vi "DIO timeline.vi"(1 "Plot?":bool[][](array[boolean]), 2 "Array":u64[][](array[numeric])=[[0, 51168, 5155], [1000, 51168, 5155], [2000, 50912, 5155], [20000, 49888, 5155], [14960, 49888, 5155], [16960, 49888, 5155], [17960, 49888, 5155], [31420, 49376, 5155], [33920, 49376, 5153], [50880, 49376, 5139], [62840, 50656, 5139], [1304, 50592, 5139], [2304, 50592, 5139], [3304, 50656, 5139], [4304, 50400, 5139], [22304, 49376, 5139], [38552, 50656, 5139], [42552, 50592, 5139], [43552, 50592, 5139], [44552, 50656, 5139], [45552, 50400, 5139], [63552, 49376, 5139], [19264, 49888, 5155], [60512, 49888, 5155], [34224, 49888, 5155], [36224, 49888, 5153], [50184, 49888, 5153], [50684, 49896, 5153], [51184, 49864, 5281], [53184, 49866, 13473], [53384, 33482, 13473], [53534, 33482, 13473], [53584, 49866, 13473], [53684, 49864, 13473], [54184, 49864, 13345], [55184, 49856, 13345], [58184, 49856, 5153], [4608, 49857, 5153], [16568, 51137, 5153], [19568, 51137, 7201], [20568, 51105, 7201], [21568, 50996, 7201], [21668, 51120, 7201], [22568, 51184, 7201], [23068, 51168, 7201], [23568, 50912, 7201], [31568, 50912, 5153], [41568, 49888, 5153], [57816, 51168, 5153], [60816, 51168, 7201], [61816, 51104, 7201], [62816, 50996, 7201], [62916, 51120, 7201], [63816, 51184, 7201], [64316, 51168, 7201], [64816, 50912, 7201], [7280, 50912, 5153], [17280, 49888, 5153], [33528, 51168, 5153], [37528, 51104, 5153], [39528, 51168, 5153], [40528, 50912, 5153], [58528, 49888, 5153], [14240, 49888, 5155]]) -> (0 "Timeline":cluster{u32[], i32[]}[](graph))   [LabVIEW 2017]
uses:
  globals/DIO board parameters global.vi
panel:
  out "Array 2":cluster{u32[], u32[]}[](array[cluster])
  # "00  01  02  03  04  05  06  07  08  09  10  11  12  13  14  15"
  # "Port A\nPort B\nPort C\nPort D"
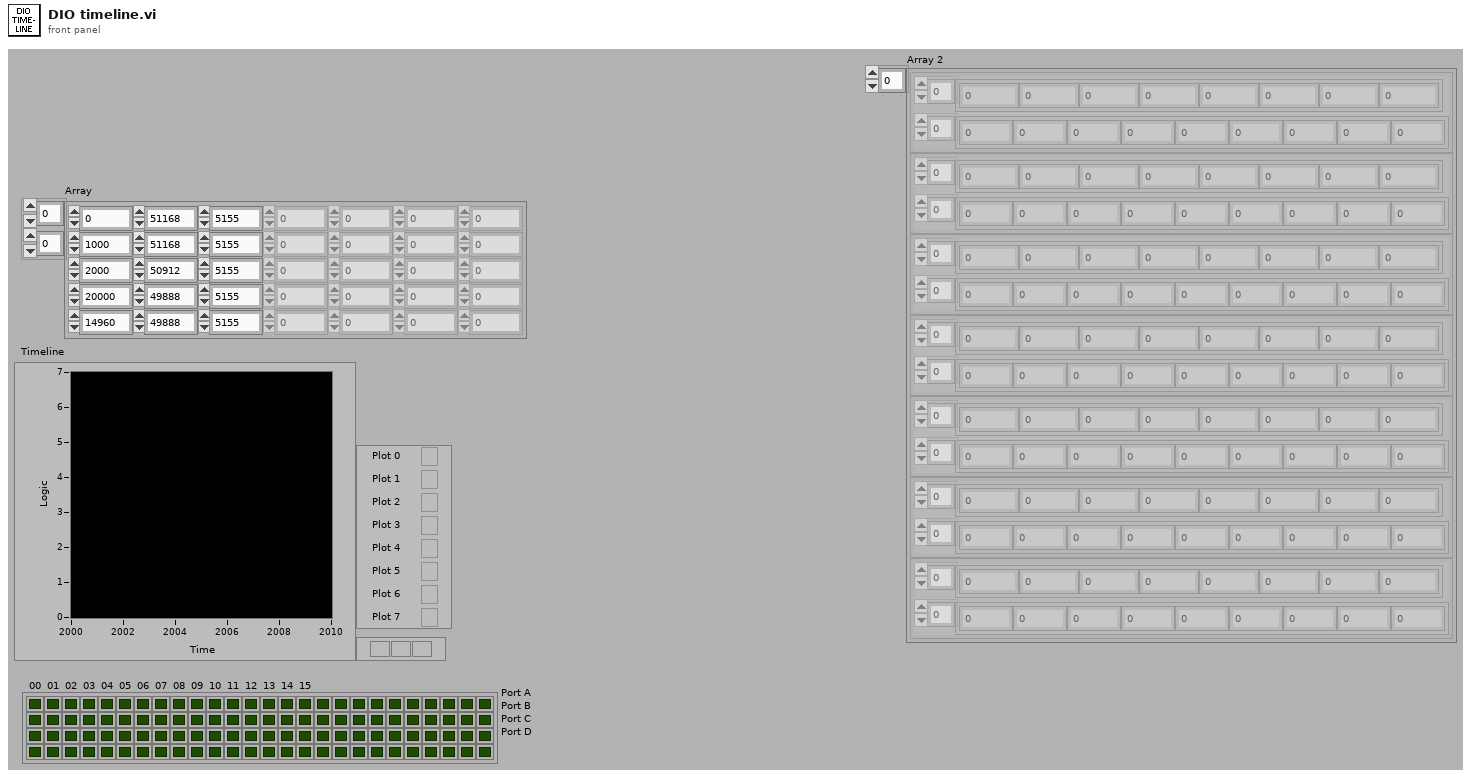
[diagram p1: front panel]
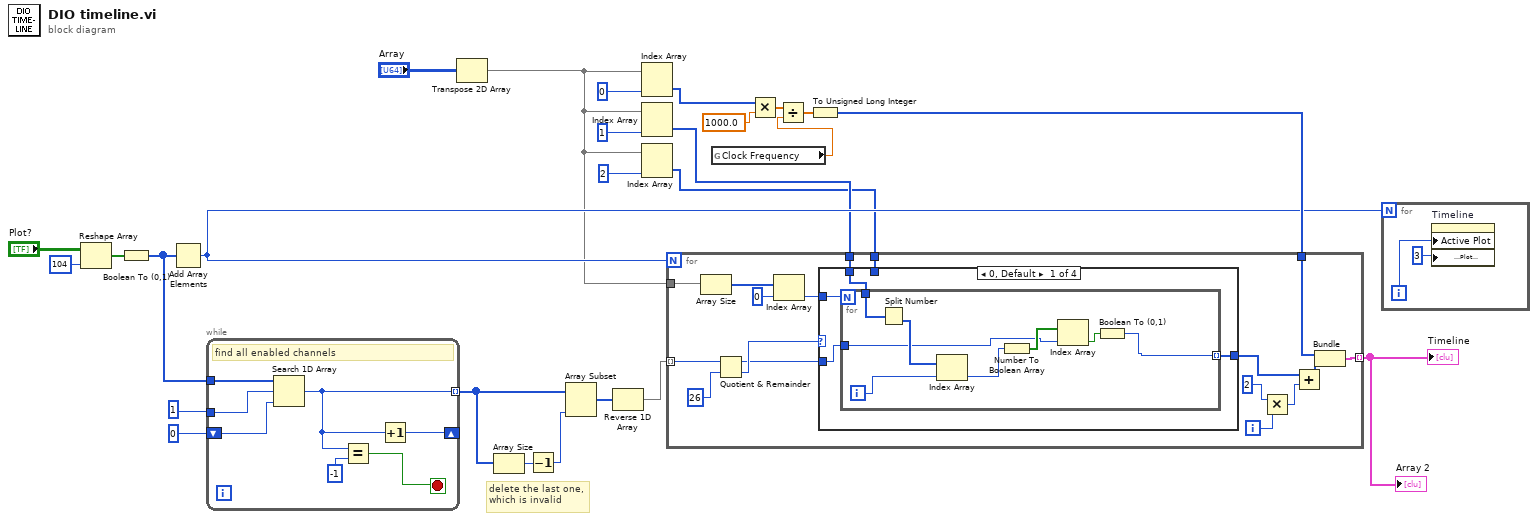
[diagram p0: block diagram]
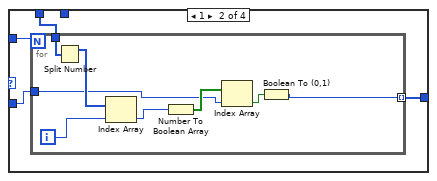
[diagram p2: hidden frame]
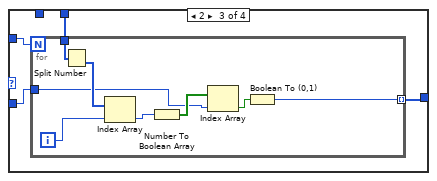
[diagram p3: hidden frame]
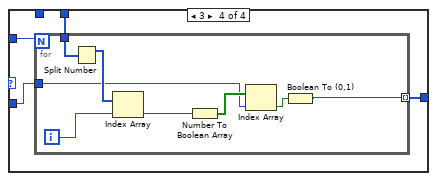
[diagram p4: hidden frame]
diagram:
  # "delete the last one,\nwhich is invalid"
  n1 = Reshape Array("Plot?", 104 ("Dimension Size")) -> (w21:bool[])
  n2 = Boolean To (0,1)(Boolean=w21) -> (0, 1=w12:i16[])
  n3 = Add Array Elements(numeric array=w12) -> (sum=w18:i16)
  n4 = while {
    tunnel: [w28] -> w15 mode=indexing
    shift-left: 0 ("index of element") -> [w30]
    shift-right: [w31] -> _
    tunnel: u32 1 ("element") -> [w32]
    tunnel: w12 -> [w33]
    stop <- w29 stop-if-true
    # "find all enabled channels"
    n5 = Search 1D Array(1D array=w33, element=w32, start index (0)=w30) -> (index of element=w28:i32)
    n6 = Equal?(x=w28, y=-1) -> (x = y?=w29:bool)
    n7 = Increment(x=w28) -> (x+1=w31:i32)
  }
  n8 = Transpose 2D Array(2D array="Array") -> (transposed array=w1:u64[][])
  n9 = Array Size(array=w15) -> (size(s)=w14:i32)
  n10 = Decrement(x=w14) -> (x-1=w13:i32)
  n11 = Array Subset(array=w15, length=w13) -> (w10:i32[])  [unwired: 1 in]
  n12 = Reverse 1D Array(array=w10) -> (reversed array=w17:i32[])
  n13 = Index Array(array=w1, index (col)=i8 0 ("Column #")) -> (element=w5:u64[])  [unwired: 1 in]
  n14 = Index Array(array=w1, index (col)=i8 1 ("Column #")) -> (element=w3:u64[])  [unwired: 1 in]
  n15 = Index Array(array=w1, index (col)=i8 2 ("Column #")) -> (element=w2:u64[])  [unwired: 1 in]
  n16 = global read "DIO board parameters global.vi" "Clock Frequency"() -> (w4:dbl)
  n17 = Multiply(x=w5, y=1000.0) -> (x*y=w25:dbl[])
  n18 = Divide(x=w25, y=w4) -> (x/y=w26:dbl[])
  n19 = To Unsigned Long Integer(number=w26) -> (unsigned 32bit integer=w20:u32[])
  n20 = for {
    N: w18 -> [_]
    tunnel: w1 -> [w48]
    tunnel: [w47] -> w19 mode=indexing
    tunnel: w17 -> [w44] mode=indexing
    tunnel: w20 -> [w46]
    tunnel: w3 -> [w42]
    tunnel: w2 -> [w41]
    i -> [w36]
    n21 = Array Size(array=w48) -> (size(s)=w50:i32[])
    n22 = Quotient & Remainder(x=w44, y=26) -> (x-y*floor(x/y)=w40:i32, floor(x/y)=w43:i32)
    n23 = Index Array(array=w50, index=0 ("Index")) -> (element=w35:i32)
    n24 = case shown="0, Default" w43 {
      tunnel: w42 -> [w53 w65 _ _]
      tunnel: w41 -> [_ _ w77 w89]
      tunnel: w40 -> [w51 w64 w76 w88]
      tunnel: w35 -> [w54 w66 w78 w90]
      tunnel: [w52 w63 w75 w87] -> w34
      frame 0, Default {
        n25 = for {
          N: w54 -> [_]
          tunnel: w53 -> [w62]
          tunnel: [w55] -> w52 mode=indexing
          tunnel: w51 -> [w56]
          i -> [w60]
          n26 = Split Number(x=w62) -> (lo(x)=w61:u32[])  [unwired: 1 out]
          n27 = Index Array(array=w61, index=w60) -> (element=w57:u32)
          n28 = Number To Boolean Array(number=w57) -> (Boolean array=w59:bool[])
          n29 = Index Array(array=w59, index=w56) -> (element=w58:bool)
          n30 = Boolean To (0,1)(Boolean=w58) -> (0, 1=w55:i16)
        }
      }
      frame 1 {
        n31 = for {
          N: w66 -> [_]
          tunnel: w65 -> [w74]
          tunnel: w64 -> [w68]
          tunnel: [w67] -> w63 mode=indexing
          i -> [w72]
          n32 = Split Number(x=w74) -> (hi(x)=w73:u32[])  [unwired: 1 out]
          n33 = Index Array(array=w73, index=w72) -> (element=w69:u32)
          n34 = Number To Boolean Array(number=w69) -> (Boolean array=w71:bool[])
          n35 = Index Array(array=w71, index=w68) -> (element=w70:bool)
          n36 = Boolean To (0,1)(Boolean=w70) -> (0, 1=w67:i16)
        }
      }
      frame 2 {
        n37 = for {
          N: w78 -> [_]
          tunnel: w77 -> [w86]
          tunnel: w76 -> [w80]
          tunnel: [w79] -> w75 mode=indexing
          i -> [w84]
          n38 = Split Number(x=w86) -> (lo(x)=w85:u32[])  [unwired: 1 out]
          n39 = Index Array(array=w85, index=w84) -> (element=w81:u32)
          n40 = Number To Boolean Array(number=w81) -> (Boolean array=w83:bool[])
          n41 = Index Array(array=w83, index=w80) -> (element=w82:bool)
          n42 = Boolean To (0,1)(Boolean=w82) -> (0, 1=w79:i16)
        }
      }
      frame 3 {
        n43 = for {
          N: w90 -> [_]
          tunnel: w89 -> [w98]
          tunnel: w88 -> [w93]
          tunnel: [w92] -> w87 mode=indexing
          i -> [w96]
          n44 = Split Number(x=w98) -> (hi(x)=w97:u32[])  [unwired: 1 out]
          n45 = Index Array(array=w97, index=w96) -> (element=w95:u32)
          n46 = Number To Boolean Array(number=w95) -> (Boolean array=w94:bool[])
          n47 = Index Array(array=w94, index=w93) -> (element=w91:bool)
          n48 = Boolean To (0,1)(Boolean=w91) -> (0, 1=w92:i16)
        }
      }
    }
    n49 = Multiply(x=2, y=w36) -> (x*y=w39:i32)
    n50 = Add(x=w34, y=w39) -> (x+y=w37:i32[])
    n51 = Bundle(w46, w37) -> (w47:cluster{u32[], i32[]})  [unwired: 1 in]
  }
  "Timeline" <- w19
  "Array 2" <- w19
  n52 = for {
    N: w18 -> [_]
    i -> [w100]
    n53 = property on="Timeline" class="XYGraph (strict)"("Active Plot"=w100, "Plot.Plot Interpolation"=u8 3) -> ()  [unwired: 2 in, 2 out]
  }
